vi "Publish to Phone Number.vi"(8 "error in (no error)":errorcluster, 10 "Message":string, 11 "Phone Number in":refnum<class "Phone Number.lvclass">) -> (0 "error out":errorcluster, 3 "Phone Number out":refnum<class "Phone Number.lvclass">)   [LabVIEW 2015, in "NI_AWS_SNS.lvlib" / "Phone Number.lvclass"]
doc: "Sends a text message (SMS message) directly to a phone number."
uses:
  Phone Number.lvclass
  Core/HTTP Request/Valid String Specification.ctl
  Core/HTTP Request/Request Options.ctl
  Core/HTTP Request/Name Value Pair.ctl
  Core/HTTP Request/Region handling.ctl
  Core/HTTP Request/URL formatting.ctl
  Phone Number.lvclass/Phone Number.ctl
  Read Phone Number.vi
  Core/HTTP Request/HTTP Request.lvclass
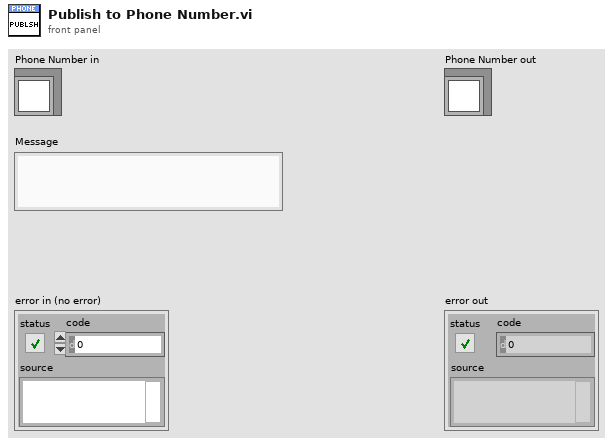
[diagram p1: front panel]
types:
  T1 = typedef "NI_AWS_Core.lvlib/HTTP Request.lvclass/Valid String Specification.ctl" = enum16{"only [alphanumeric][-][_]", "phone number +1xxxyyyzzzz"}
  T2 = typedef "NI_AWS_Core.lvlib/HTTP Request.lvclass/Name Value Pair.ctl" = cluster{"name":string, "value":string}
  T3 = typedef "NI_AWS_Core.lvlib/HTTP Request.lvclass/Request Options.ctl" = cluster{"request headers":T2[], "request parameters":T2[], "request body":string, "region handling":T4, "URL formatting":T5}
  T4 = typedef "NI_AWS_Core.lvlib/HTTP Request.lvclass/Region handling.ctl" = enum16{"use region everywhere", "use region (authentication only)", "use region (URL only)", "ignore region everwhere"}
  T5 = typedef "NI_AWS_Core.lvlib/HTTP Request.lvclass/URL formatting.ctl" = enum16{"region-", "region."}
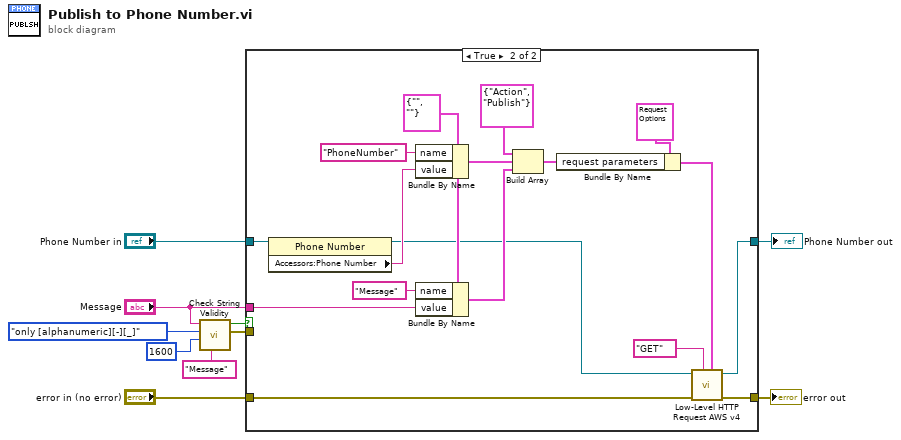
[diagram p0: block diagram]
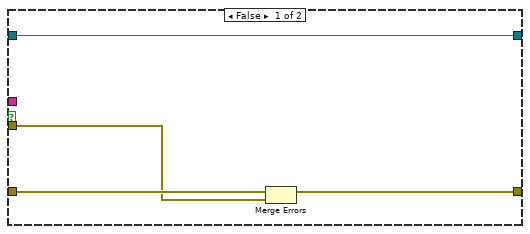
[diagram p2: hidden frame]
diagram:
  n1 = call "Check String Validity.vi"("String Name for Error"="Message", "Max Characters"=1600, "Valid String Specification"=Valid_String_Specification."only [alphanumeric][-][_]", "String"="Message") -> ("string error"=w5:errorcluster, "Valid"=w6:bool)  [unwired: 6 in]
  n2 = case shown="True" w6 {
    tunnel: "error in (no error)" -> [w13 w31]
    tunnel: [w12 w30] -> w9
    tunnel: "Phone Number in" -> [w14 w24]
    tunnel: "Message" -> [_ w20]
    tunnel: w5 -> [w11 _]
    tunnel: [w14 w16] -> w1
    frame False {
      n3 = Merge Errors(w13, w11) -> (w12:errorcluster)
    }
    frame True {
      w22 = T2 {"name"="", "value"=""} ("Name Value Pair")
      n4 = property class="Phone Number"(reference=w24) -> (reference out=w15:refnum<class "Phone Number.lvclass">, "Accessors:Phone Number"=w23:string)  [unwired: 1 in, 1 out]
      n5 = Bundle By Name(cluster=w22, "name"="PhoneNumber", "value"=w23) -> (w26:T2)
      n6 = Bundle By Name(cluster=w22, "name"="Message", "value"=w20) -> (w19:T2)
      n7 = Build Array(T2 {"name"="Action", "value"="Publish"} ("Name Value Pair"), w26, w19) -> (w28:T2[])
      n8 = Bundle By Name(cluster=T3 {"request headers"=[], "request parameters"=[{"name"="Action", "value"="ListQueues"}], "request body"="", "region handling"=enum."use region everywhere", "URL formatting"=enum."region."} ("Request Options"), "request parameters"=w28) -> (w17:T3)
      n9 = call "Low-Level HTTP Request AWS v4.vi"("Request Options"=w17, "HTTP-Verb"="GET", "error in (no error)"=w31, "AWS Core in"=w15) -> ("error out"=w30:errorcluster, "AWS Core out"=w16:refnum<class "Phone Number.lvclass">)  [unwired: 4 in, 2 out]
    }
  }
  "error out" <- w9
  "Phone Number out" <- w1
